vi "疫苗信息检索.vi"(1 "疫苗编号":i32, 2 "connection reference":T1) -> (0 "疫苗数据":T2 {"生产日期" format="%<%Y/%m/%d>T"})   [LabVIEW 2018]
uses:
  <vilib>/addons/database/Connection.llb/Conn ObjectReference.ctl
  <vilib>/addons/database/_DB Variant To Data/Database Variant To Data.xnode
  <vilib>/addons/database/NI_Database_API.lvlib
panel:
  out "error out":errorcluster caption="错误输出"
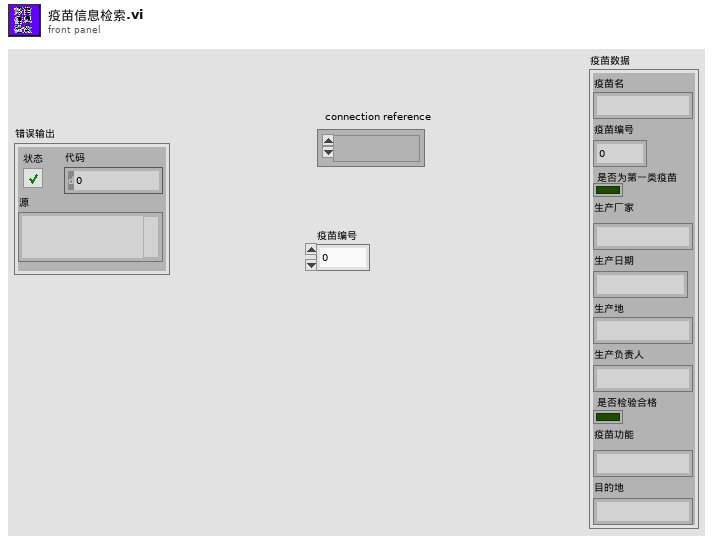
[diagram p1: front panel]
types:
  T1 = typedef "NI_Database_API.lvlib/Conn ObjectReference.ctl" = refnum<k1>
  T2 = typedef "疫苗信息.ctl" = cluster{"疫苗名":string, "疫苗编号":i32, "是否为第一类疫苗":bool, "生产厂家":string, "生产日期":timestamp, "生产地":string, "生产负责人":string, "是否检验合格":bool, "疫苗功能":string, "目的地":string}
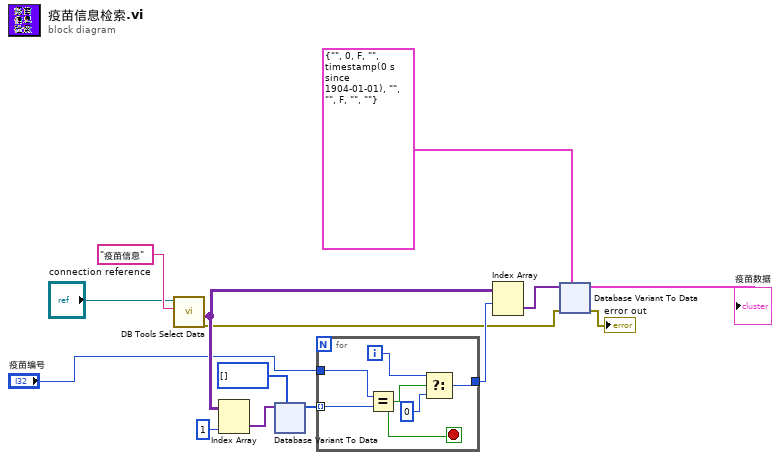
[diagram p0: block diagram]
diagram:
  n1 = call <vilib>:"DB Tools Select Data.vi"("table"="疫苗信息", "connection reference"="connection reference") -> ("error out"=w2:errorcluster, "data"=w9:variant[][])  [unwired: 4 in, 1 out]
  n2 = Index Array(array=w9, index (col)=1 ("禁用的索引 (列)")) -> (element=w12:variant[])  [unwired: 1 in]
  n3 = xnode "Database Variant To Data"("database variant"=w12, "type"=i32[] []) -> ("data"=w10:i32[])  [unwired: 1 in, 1 out]
  n4 = for {
    tunnel: w10 -> [w19] mode=indexing
    tunnel: "疫苗编号" -> [w20]
    tunnel: [w18] -> w8
    i -> [w16]
    stop <- w17 stop-if-true
    n5 = Equal?(x=w20, y=w19) -> (x = y?=w17:bool)
    n6 = Select(t=w16, s=w17, f=0) -> (s? t:f=w18:i32)
  }
  n7 = Index Array(array=w9, index (row)=w8) -> (element=w7:variant[])  [unwired: 1 in]
  n8 = xnode "Database Variant To Data"("database variant"=w7, "error in (no error)"=w2, "type"=T2 {"疫苗名"="", "疫苗编号"=0, "是否为第一类疫苗"=FALSE, "生产厂家"="", "生产日期"=timestamp(0 s since 1904-01-01), "生产地"="", "生产负责人"="", "是否检验合格"=FALSE, "疫苗功能"="", "目的地"=""} ("簇")) -> ("data"=→"疫苗数据":T2, "error out"=→"error out":errorcluster)
